vi "Generate Error Cluster.vi"(8 "error in (no error)":errorcluster, 9 "Additional Message":string, 11 "Code":i32) -> (0 "error out":errorcluster)   [LabVIEW 2017, in "NI_XML.lvlib"]
uses:
  <vilib>/xml/NI_XML.lvlib
panel:
  in  "XML DOM Parser":string="XML Parser reported the following"
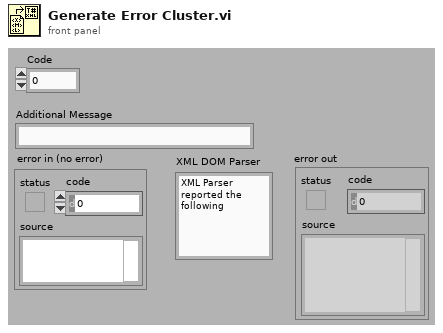
[diagram p1: front panel]
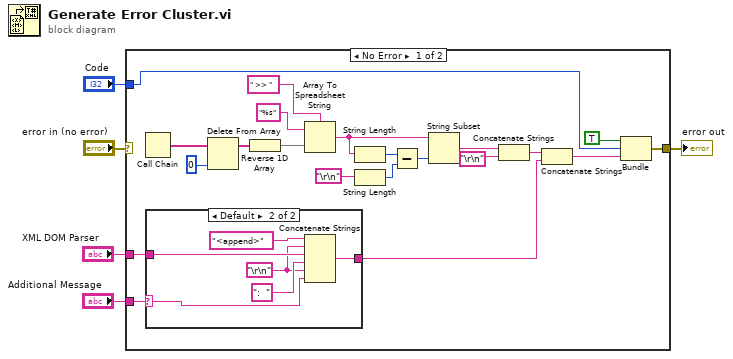
[diagram p0: block diagram]
diagram:
  n1 = case shown="No Error" "error in (no error)" {
    selector: "error in (no error)" -> [_ w34]
    tunnel: [w26 w34] -> w4
    tunnel: "Code" -> [w8 _]
    tunnel: "Additional Message" -> [w7 _]
    tunnel: "XML DOM Parser" -> [w6 _]
    frame No Error {
      n2 = Call Chain() -> (call chain=w17:string[])
      n3 = case shown="Default" w7 {
        selector: w7 -> [w27 w30]
        tunnel: [w27 w33] -> w21
        tunnel: w6 -> [_ w32]
        frame "" {
        }
        frame Default {
          w28 = "\r\n"
          n4 = Concatenate Strings("<append>", w28, w32, ":  " ("string"), w28, w30) -> (w33:string)
        }
      }
      n5 = Delete From Array(array=w17, index=0 ("Index")) -> (array with subset deleted=w12:string[])  [unwired: 1 in, 1 out]
      n6 = Reverse 1D Array(array=w12) -> (reversed array=w14:string[])
      n7 = Array To Spreadsheet String(delimiter (Tab)=" >> ", array=w14, 3:"%s" ("format string")) -> (spreadsheet string=w11:string)
      n8 = String Length(string=w11) -> (length=w15:i32)
      n9 = String Length(string="\r\n") -> (length=w9:i32)
      n10 = Subtract(x=w15, y=w9) -> (x-y=w16:i32)
      n11 = String Subset(string=w11, length (rest)=w16) -> (substring=w22:string)  [unwired: 1 out]
      n12 = Concatenate Strings(w22, "\r\n") -> (w23:string)
      n13 = Concatenate Strings(w23, w21) -> (w24:string)
      n14 = Bundle(TRUE, "Code"=w8, w24) -> (w26:cluster{bool, "Code":i32, string})  [unwired: 1 out]
    }
    frame Error {
      # "Cluster already contains error"
    }
  }
  "error out" <- w4
